vi "SSL Detection Robots Delete Invalids Kalman.vi"(5 "Now":timestamp, 7 "Life Time":dbl=1.0, 11 "Robots In":T3(array[cluster]) {"Detection Robot"."height" format="%+4.3f"; "Detection Robot"."pixel_y" format="%+4.3f"; "Detection Robot"."pixel_x" format="%+4.3f"; "Detection Robot"."orientation" format="%+4.3f"; "Detection Robot"."y" format="%+4.3f"; "Detection Robot"."confidence" format="%4.3f"; "Detection Robot"."x" format="%+4.3f"}) -> (3 "Robots Out":T3(array[cluster]) {"Detection Robot"."height" format="%+4.3f"; "Detection Robot"."pixel_y" format="%+4.3f"; "Detection Robot"."pixel_x" format="%+4.3f"; "Detection Robot"."orientation" format="%+4.3f"; "Detection Robot"."y" format="%+4.3f"; "Detection Robot"."confidence" format="%4.3f"; "Detection Robot"."x" format="%+4.3f"})   [LabVIEW 2016]
uses:
  SSL Detection Robot.ctl
  <vilib>/Analysis/Matrix/Datatypes/RealMatrix.ctl
  <vilib>/Analysis/Matrix/NI_Matrix.lvlib
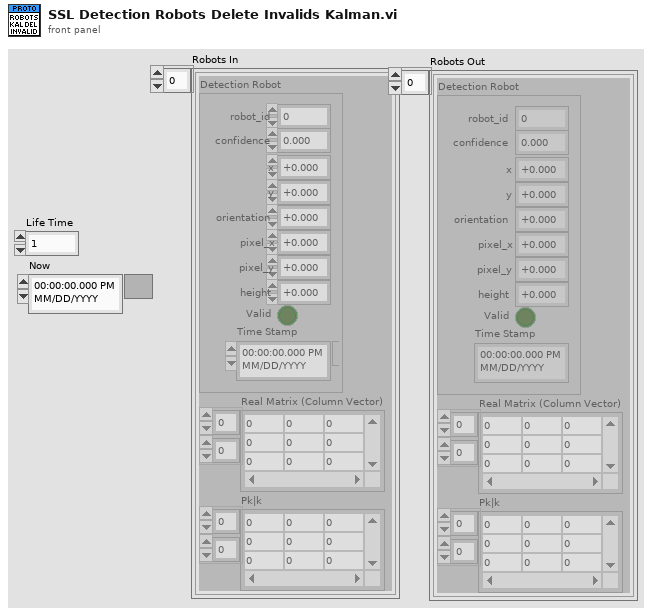
[diagram p1: front panel]
types:
  T1 = typedef "SSL Detection Robot.ctl" = cluster{"x":sgl, "robot_id":u32, "confidence":sgl, "y":sgl, "orientation":sgl, "pixel_x":sgl, "pixel_y":sgl, "height":sgl, "Valid":bool, "Time Stamp":timestamp}
  T2 = typedef "NI_Matrix.lvlib/RealMatrix.ctl" = dbl[][]
  T3 = cluster{"Detection Robot":T1, "Real Matrix (Column Vector)":T2, "Pk|k":T2}[]
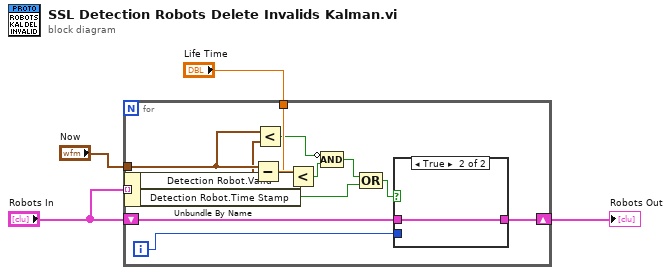
[diagram p0: block diagram]
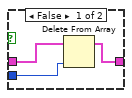
[diagram p2: hidden frame]
diagram:
  n1 = for {
    tunnel: "Robots In" -> [w17] mode=indexing
    shift-right: [w14] -> w1
    shift-left: "Robots In" -> [w16]
    tunnel: "Now" -> [w9]
    tunnel: "Life Time" -> [w12]
    i -> [w15]
    n2 = Unbundle By Name(w17) -> ("Detection Robot.Valid"=w11:bool, "Detection Robot.Time Stamp"=w8:timestamp)
    n3 = Subtract(x=w9, y=w8) -> (x-y=w13:dbl)
    n4 = Less?(x=w9, y=w8) -> (x < y?=w7:bool)
    n5 = Less?(x=w13, y=w12) -> (x < y?=w6:bool)
    n6 = Compound Arithmetic op=AND(invert w7, w6) -> (w5:bool)
    n7 = Compound Arithmetic op=OR(w5, w11) -> (w10:bool)
    n8 = case shown="True" w10 {
      tunnel: w16 -> [w20 w21]
      tunnel: w15 -> [w19 _]
      tunnel: [w18 w21] -> w14
      frame False {
        n9 = Delete From Array(array=w20, index=w19) -> (array with subset deleted=w18:T3)  [unwired: 1 in, 1 out]
      }
      frame True {
      }
    }
  }
  "Robots Out" <- w1
